vi "get_value_from_archive.vi"(9 "channel":string="channel", 10 "group":string="channel", 11 "archive":T1={"sync"={"elyse/sync/NI6071E/delay"=1.5500000000000005, "elyse/sync/NI6071E/width"=1.0, "elyse/sync/frequency/delay"=10.0, "elyse/sync/frequency/width"=181000.0, "elyse/sync/WCM/delay"=2177.9, "elyse/sync/WCM/width"=10.0, "elyse/sync/modulator/delay"=2182.400000000002, "elyse/sync/modulator/width"=3.0, "elyse/sync/HF/delay"=2175.0, "elyse/sync/HF/width"=3.0, "elyse/sync/Faraday/delay"=5080.0, "elyse/sync/Faraday/width"=100.0, "elyse/sync/Oscilloscope/delay"=2175.0, "elyse/sync/Oscilloscope/width"=2.8, "elyse/sync/50Hz_20MHz/delay"=1.0, "elyse/sync/50Hz_20MHz/width"=5000.0, "elyse/sync/laser_HF/delay"=0.35, "elyse/sync/laser_HF/width"=0.35, "elyse/sync/IMAC/delay"=2176.0, "elyse/sync/IMAC/width"=100.0, "elyse/sync/laser/delay"=2008.3, "elyse/sync/laser/width"=10.0, "elyse/sync/oscilloscope1/delay"=2175.0, "elyse/sync/oscilloscope1/width"=10.0, "elyse/sync/oscilloscope2/delay"=2175.0, "elyse/sync/oscilloscope2/width"=100.0, "elyse/sync/detection1/delay"=500.0, "elyse/sync/detection1/width"=500.0, "elyse/sync/detection1/delay"=0.3, "elyse/sync/detection2/width"=10.0, "elyse/sync/machine/delay"=2175.0, "elyse/sync/machine/width"=100.0, "elyse/sync/n_selection"=4.0}, "HT"={"elyse/HT/voltage/set_value"=6.5, "elyse/HT/voltage/value"=1.5625e-08, "elyse/HT/current/value"=0.0, "elyse/preamplifier/set_value"=1.5625e-08, "elyse/preamplifier/value"=0.0}, "HF"={"elyse/HF/attenuator/value"=-0.01903046052094623, "elyse/HF/dephaser/value"=-18.585806237727724, "elyse/HF/dephaser/value_manuel"=-78.82860725035081, "elyse/HF/canon/value"=0.0, "elyse/HF/section/value"=-18.585806237727724}, "vacuum"={"elyse/vacuum/preparation_chamber/state"=TRUE, "elyse/vacuum/preparation_chamber/measurement"=0.0, "elyse/vacuum/HF/state"=TRUE, "elyse/vacuum/HF/measurement"=0.0, "elyse/vacuum/canon/state"=TRUE, "elyse/vacuum/canon/measurement"=0.0, "elyse/vacuum/section/state"=TRUE, "elyse/vacuum/section/measurement"=0.0, "elyse/vacuum/dipole1/state"=TRUE, "elyse/vacuum/dipole1/measurement"=0.0, "elyse/vacuum/screen1/state"=TRUE, "elyse/vacuum/screen1/measurement"=0.0, "elyse/vacuum/mirror/state"=TRUE, "elyse/vacuum/mirror/measurement"=0.0, "elyse/vacuum/tpg300_section/state"=TRUE, "elyse/vacuum/tpg300_section/measurement"=0.0, "elyse/vacuum/valves/cathode/state"=FALSE, "elyse/vacuum/valves/injection/state"=FALSE}, "modulator"={"elyse/modulator/focale1/current/value"=0.0, "elyse/modulator/focale2/current/value"=0.0, "elyse/modulator/focale3/current/value"=0.0, "elyse/modulator/LAR/voltage/value"=0.0, "elyse/modulator/line_end/current/value"=0.0, "elyse/modulator/thyratron/currents/power/value"=0.0, "elyse/modulator/thyratron_reservoir/current/value"=0.0, "elyse/modulator/paramagnetization/current/value"=0.0, "elyse/modulator/thyratron/voltages/heating/value"=0.0, "elyse/modulator/thyratron/currents/heating/value"=0.0, "elyse/modulator/klystron/currents/power/value"=0.0, "elyse/modulator/klystron/voltages/power/value"=0.0, "elyse/modulator/klystron/currents/heating/value"=0.0, "elyse/modulator/klystron/voltages/heating/value"=0.0}, "cooling"={"elyse/cooling/section/temperature/set_value"=28.0, "elyse/cooling/section/temperature/measurement"=27.96142578125, "elyse/cooling/canon/temperature/set_value"=20.2, "elyse/cooling/canon/temperature/measurement"=26.69921875}, "magnets"={"elyse/magnets/focale/set_value"=0.0, "elyse/magnets/focale/value"=0.0, "elyse/magnets/phase_HF_laser/set_value"=0.0, "elyse/magnets/phase_HF_laser/value"=0.0, "elyse/magnets/dipole1/set_value"=0.0, "elyse/magnets/dipole1/value"=0.0, "elyse/magnets/dipole2/set_value"=0.0, "elyse/magnets/dipole2/value"=0.0, "elyse/magnets/Cor_H1/set_value"=0.0, "elyse/magnets/Cor_H1/value"=0.0, "elyse/magnets/Cor_V1/set_value"=0.0, "elyse/magnets/Cor_V1/value"=0.0, "elyse/magnets/Cor_H2/set_value"=0.0, "elyse/magnets/Cor_H2/value"=0.0, "elyse/magnets/Cor_V2/set_value"=0.0, "elyse/magnets/Cor_V2/value"=0.0, "elyse/magnets/Cor_H3/set_value"=0.0, "elyse/magnets/Cor_H3/value"=0.0, "elyse/magnets/Cor_V3/set_value"=-5.0, "elyse/magnets/Cor_V3/value"=0.0, "elyse/magnets/Cor_H4/set_value"=0.0, "elyse/magnets/Cor_H4/value"=0.0, "elyse/magnets/Cor_V4/set_value"=0.0, "elyse/magnets/Cor_V4/value"=0.0, "elyse/magnets/Cor_H5/set_value"=0.0, "elyse/magnets/Cor_H5/value"=0.0, "elyse/magnets/Cor_V5/set_value"=0.0, "elyse/magnets/Cor_V5/value"=0.0, "elyse/magnets/triplet1-1/set_value"=0.0, "elyse/magnets/triplet1-1/value"=0.0, "elyse/magnets/triplet1-2/set_value"=0.0, "elyse/magnets/triplet1-2/value"=0.0, "elyse/magnets/triplet2-1/set_value"=0.0, "elyse/magnets/triplet2-1/value"=0.0, "elyse/magnets/triplet2-2/set_value"=0.0, "elyse/magnets/triplet2-2/value"=0.0, "elyse/magnets/qudrupole1/set_value"=0.0, "elyse/magnets/qudrupole1/value"=0.0, "elyse/magnets/qudrupole2/set_value"=0.0, "elyse/magnets/qudrupole2/value"=0.0}, "time"={"elyse/timestamp"=0.0}}) -> (3 "value":dbl)   [LabVIEW 2020]
uses:
  archive.ctl
  sync_type_def.ctl
  HT_type-def.ctl
  HF_type_def.ctl
  vacuum_type_def.ctl
  modulator_type_def.ctl
  water_cooling_type_def.ctl
  all_magnets_type_def.ctl
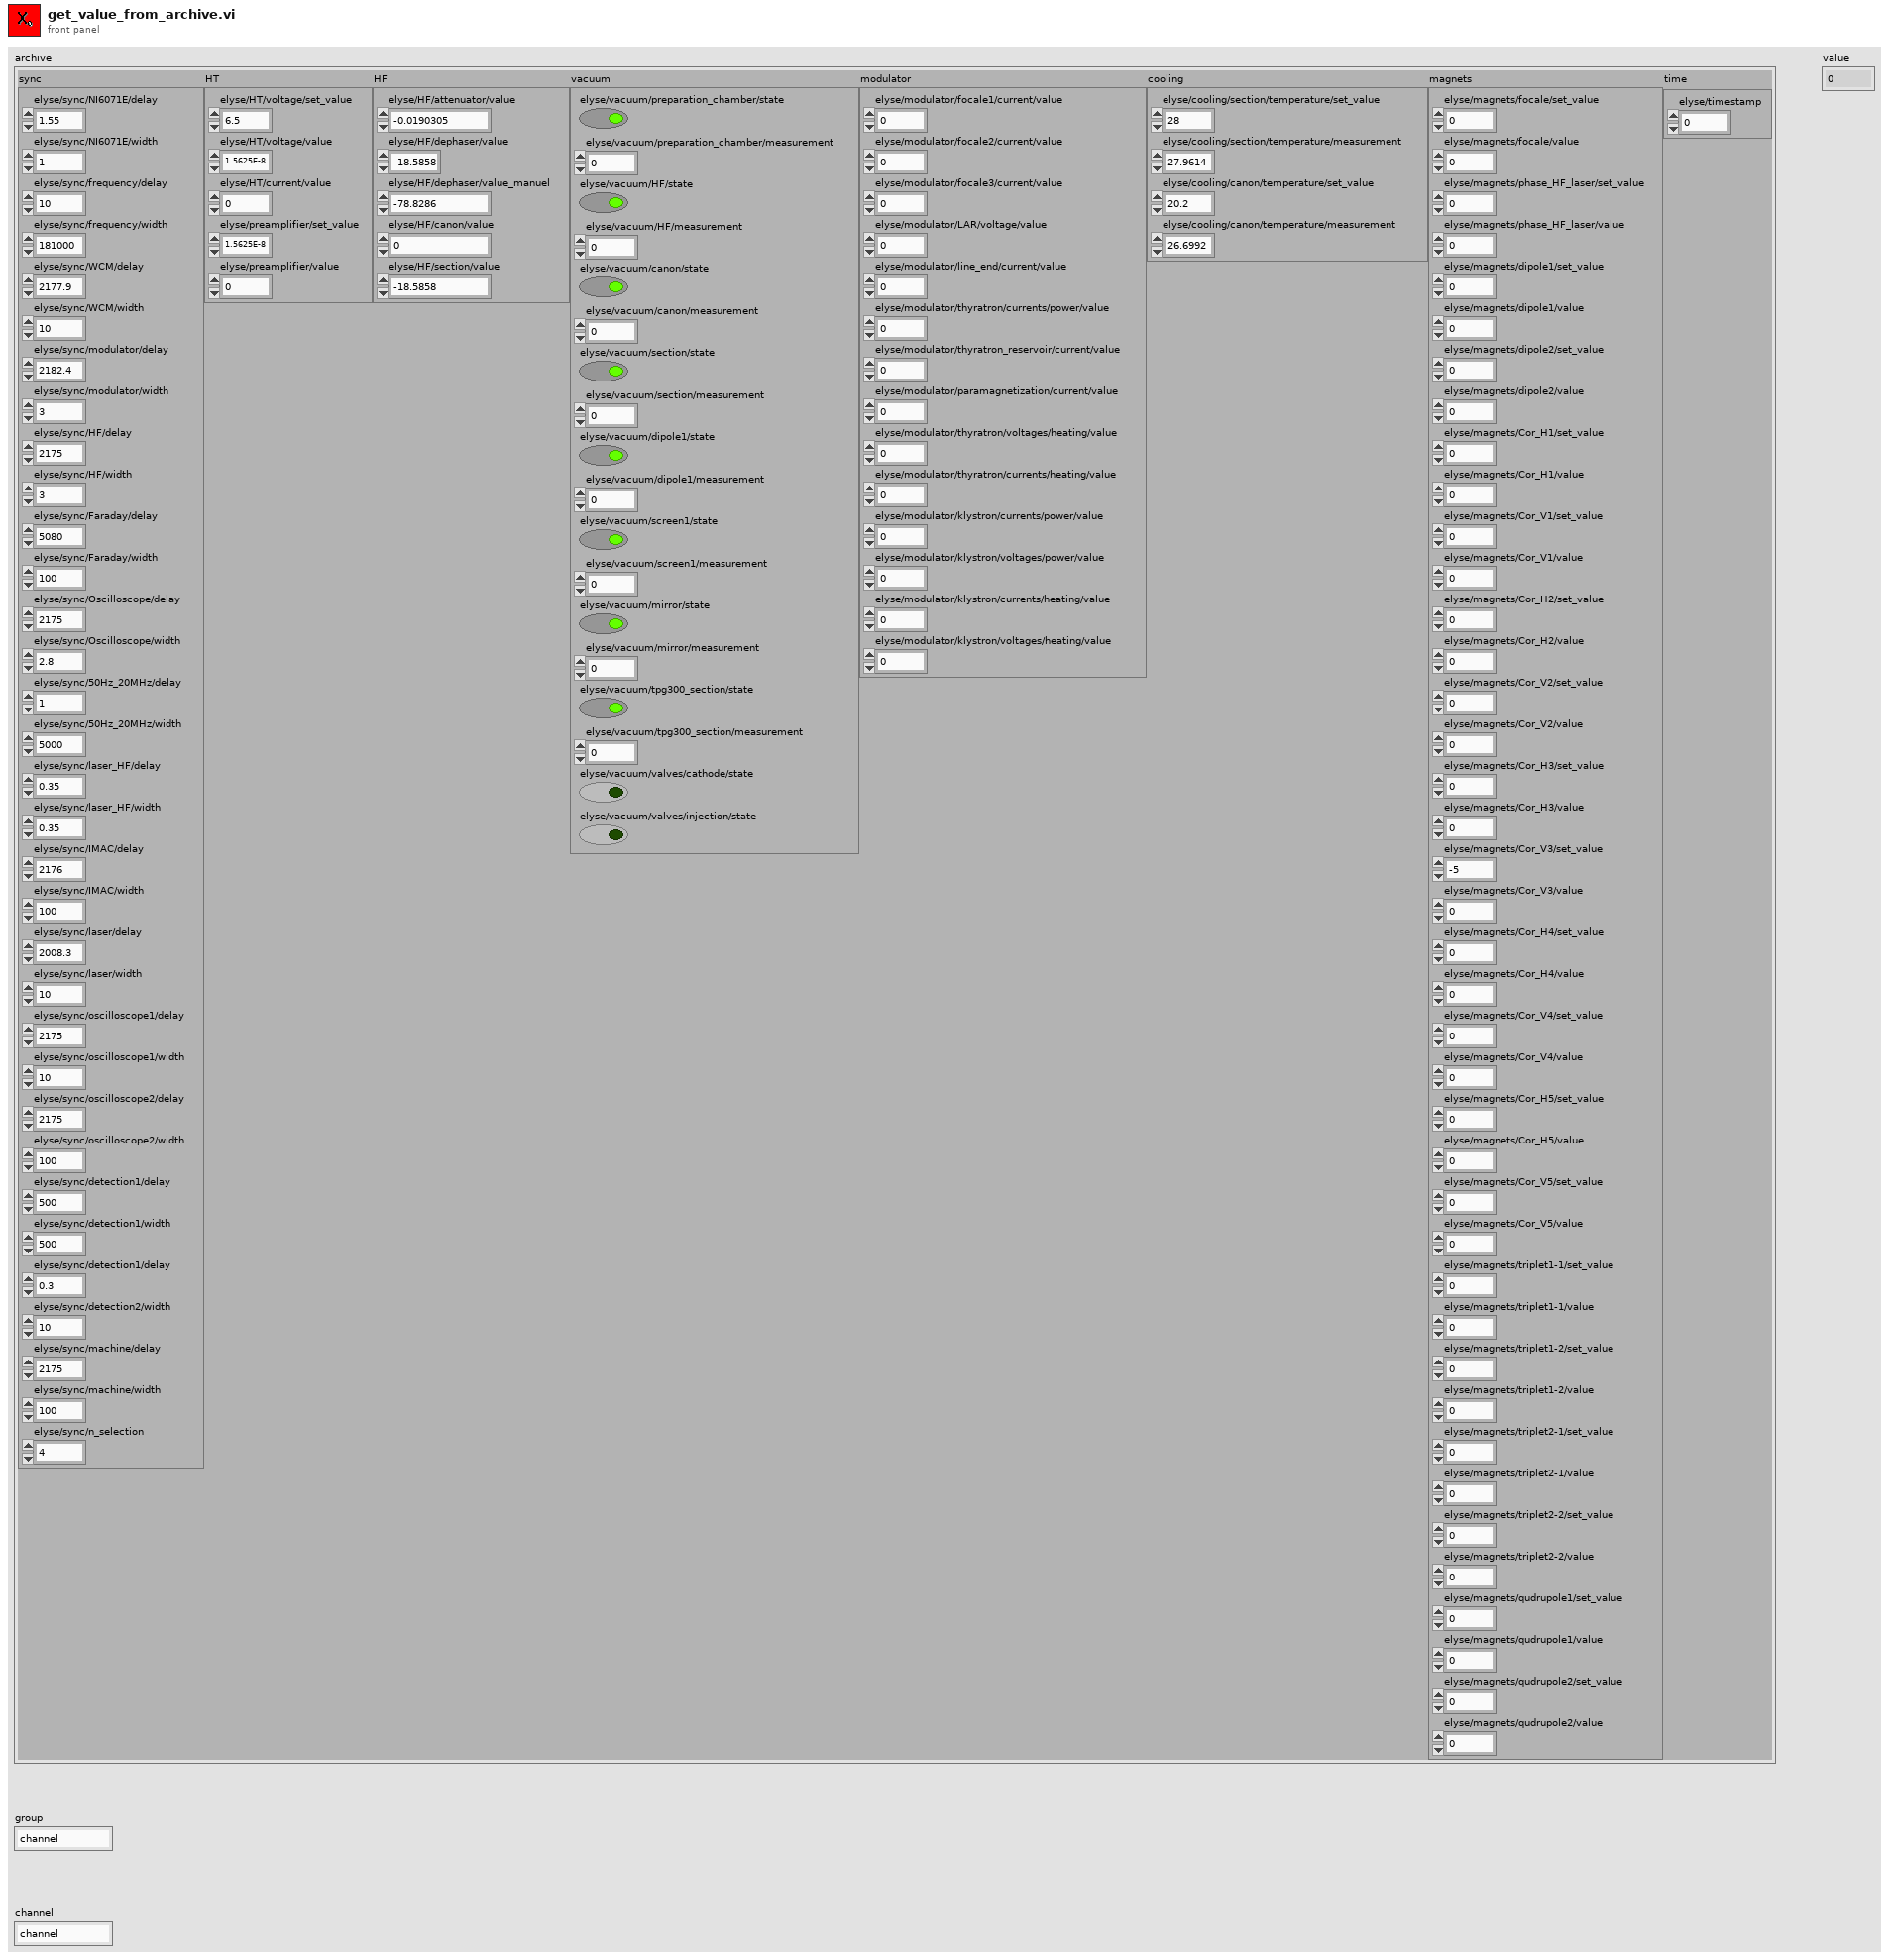
[diagram p1: front panel]
types:
  T1 = typedef "archive.ctl" = cluster{"sync":T2, "HT":T3, "HF":T4, "vacuum":T5, "modulator":T6, "cooling":T7, "magnets":T8, "time":cluster{"elyse/timestamp":dbl}}
  T2 = typedef "sync_type_def.ctl" = cluster{"elyse/sync/NI6071E/delay":dbl, "elyse/sync/NI6071E/width":dbl, "elyse/sync/frequency/delay":dbl, "elyse/sync/frequency/width":dbl, "elyse/sync/WCM/delay":dbl, "elyse/sync/WCM/width":dbl, "elyse/sync/modulator/delay":dbl, "elyse/sync/modulator/width":dbl, "elyse/sync/HF/delay":dbl, "elyse/sync/HF/width":dbl, "elyse/sync/Faraday/delay":dbl, "elyse/sync/Faraday/width":dbl, "elyse/sync/Oscilloscope/delay":dbl, "elyse/sync/Oscilloscope/width":dbl, "elyse/sync/50Hz_20MHz/delay":dbl, "elyse/sync/50Hz_20MHz/width":dbl, "elyse/sync/laser_HF/delay":dbl, "elyse/sync/laser_HF/width":dbl, "elyse/sync/IMAC/delay":dbl, "elyse/sync/IMAC/width":dbl, "elyse/sync/laser/delay":dbl, "elyse/sync/laser/width":dbl, "elyse/sync/oscilloscope1/delay":dbl, "elyse/sync/oscilloscope1/width":dbl, "elyse/sync/oscilloscope2/delay":dbl, "elyse/sync/oscilloscope2/width":dbl, "elyse/sync/detection1/delay":dbl, "elyse/sync/detection1/width":dbl, "elyse/sync/detection1/delay":dbl, "elyse/sync/detection2/width":dbl, "elyse/sync/machine/delay":dbl, "elyse/sync/machine/width":dbl, "elyse/sync/n_selection":dbl}
  T3 = typedef "HT_type-def.ctl" = cluster{"elyse/HT/voltage/set_value":dbl, "elyse/HT/voltage/value":dbl, "elyse/HT/current/value":dbl, "elyse/preamplifier/set_value":dbl, "elyse/preamplifier/value":dbl}
  T4 = typedef "HF_type_def.ctl" = cluster{"elyse/HF/attenuator/value":dbl, "elyse/HF/dephaser/value":dbl, "elyse/HF/dephaser/value_manuel":dbl, "elyse/HF/canon/value":dbl, "elyse/HF/section/value":dbl}
  T5 = typedef "vacuum_type_def.ctl" = cluster{"elyse/vacuum/preparation_chamber/state":bool, "elyse/vacuum/preparation_chamber/measurement":dbl, "elyse/vacuum/HF/state":bool, "elyse/vacuum/HF/measurement":dbl, "elyse/vacuum/canon/state":bool, "elyse/vacuum/canon/measurement":dbl, "elyse/vacuum/section/state":bool, "elyse/vacuum/section/measurement":dbl, "elyse/vacuum/dipole1/state":bool, "elyse/vacuum/dipole1/measurement":dbl, "elyse/vacuum/screen1/state":bool, "elyse/vacuum/screen1/measurement":dbl, "elyse/vacuum/mirror/state":bool, "elyse/vacuum/mirror/measurement":dbl, "elyse/vacuum/tpg300_section/state":bool, "elyse/vacuum/tpg300_section/measurement":dbl, "elyse/vacuum/valves/cathode/state":bool, "elyse/vacuum/valves/injection/state":bool}
  T6 = typedef "modulator_type_def.ctl" = cluster{"elyse/modulator/focale1/current/value":dbl, "elyse/modulator/focale2/current/value":dbl, "elyse/modulator/focale3/current/value":dbl, "elyse/modulator/LAR/voltage/value":dbl, "elyse/modulator/line_end/current/value":dbl, "elyse/modulator/thyratron/currents/power/value":dbl, "elyse/modulator/thyratron_reservoir/current/value":dbl, "elyse/modulator/paramagnetization/current/value":dbl, "elyse/modulator/thyratron/voltages/heating/value":dbl, "elyse/modulator/thyratron/currents/heating/value":dbl, "elyse/modulator/klystron/currents/power/value":dbl, "elyse/modulator/klystron/voltages/power/value":dbl, "elyse/modulator/klystron/currents/heating/value":dbl, "elyse/modulator/klystron/voltages/heating/value":dbl}
  T7 = typedef "water_cooling_type_def.ctl" = cluster{"elyse/cooling/section/temperature/set_value":dbl, "elyse/cooling/section/temperature/measurement":dbl, "elyse/cooling/canon/temperature/set_value":dbl, "elyse/cooling/canon/temperature/measurement":dbl}
  T8 = typedef "all_magnets_type_def.ctl" = cluster{"elyse/magnets/focale/set_value":dbl, "elyse/magnets/focale/value":dbl, "elyse/magnets/phase_HF_laser/set_value":dbl, "elyse/magnets/phase_HF_laser/value":dbl, "elyse/magnets/dipole1/set_value":dbl, "elyse/magnets/dipole1/value":dbl, "elyse/magnets/dipole2/set_value":dbl, "elyse/magnets/dipole2/value":dbl, "elyse/magnets/Cor_H1/set_value":dbl, "elyse/magnets/Cor_H1/value":dbl, "elyse/magnets/Cor_V1/set_value":dbl, "elyse/magnets/Cor_V1/value":dbl, "elyse/magnets/Cor_H2/set_value":dbl, "elyse/magnets/Cor_H2/value":dbl, "elyse/magnets/Cor_V2/set_value":dbl, "elyse/magnets/Cor_V2/value":dbl, "elyse/magnets/Cor_H3/set_value":dbl, "elyse/magnets/Cor_H3/value":dbl, "elyse/magnets/Cor_V3/set_value":dbl, "elyse/magnets/Cor_V3/value":dbl, "elyse/magnets/Cor_H4/set_value":dbl, "elyse/magnets/Cor_H4/value":dbl, "elyse/magnets/Cor_V4/set_value":dbl, "elyse/magnets/Cor_V4/value":dbl, "elyse/magnets/Cor_H5/set_value":dbl, "elyse/magnets/Cor_H5/value":dbl, "elyse/magnets/Cor_V5/set_value":dbl, "elyse/magnets/Cor_V5/value":dbl, "elyse/magnets/triplet1-1/set_value":dbl, "elyse/magnets/triplet1-1/value":dbl, "elyse/magnets/triplet1-2/set_value":dbl, "elyse/magnets/triplet1-2/value":dbl, "elyse/magnets/triplet2-1/set_value":dbl, "elyse/magnets/triplet2-1/value":dbl, "elyse/magnets/triplet2-2/set_value":dbl, "elyse/magnets/triplet2-2/value":dbl, "elyse/magnets/qudrupole1/set_value":dbl, "elyse/magnets/qudrupole1/value":dbl, "elyse/magnets/qudrupole2/set_value":dbl, "elyse/magnets/qudrupole2/value":dbl}
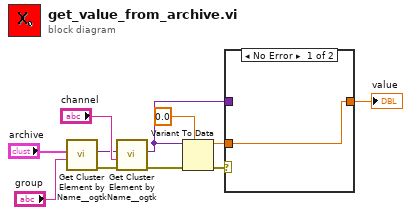
[diagram p0: block diagram]
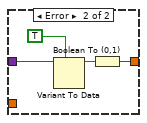
[diagram p2: hidden frame]
diagram:
  n1 = call <userlib>:"Get Cluster Element by Name__ogtk.vi"("Element Name"="group", "Cluster"="archive") -> ("error out"=w1:errorcluster, "VElement"=w8:variant)  [unwired: 7 in, 1 out]
  n2 = call <userlib>:"Get Cluster Element by Name__ogtk.vi"("error in (no error)"=w1, "Element Name"="channel", "Cluster"=w8) -> ("error out"=w2:errorcluster, "VElement"=w3:variant)  [unwired: 6 in, 1 out]
  n3 = Variant To Data(error in=w2, type=0.0, Variant=w3) -> (data=w4:dbl, error out=w6:errorcluster)
  n4 = case shown="No Error" w6 {
    tunnel: [w12 w14] -> w5
    tunnel: w4 -> [w12 _]
    tunnel: w3 -> [_ w13]
    frame No Error {
    }
    frame Error {
      n5 = Variant To Data(type=TRUE, Variant=w13) -> (data=w15:bool)  [unwired: 1 in, 1 out]
      n6 = Boolean To (0,1)(Boolean=w15) -> (0, 1=w14:i16)
    }
  }
  "value" <- w5
